vi "Persistent Data to XML.vi"() -> (0 "XML Data":string)   [LabVIEW 2013]
uses:
  Types/Persistent Data.ctl
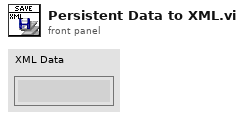
[diagram p1: front panel]
types:
  T1 = typedef "Persistent Data.ctl" = cluster{"File Name":string, "Save Directory":path, "Version":string}
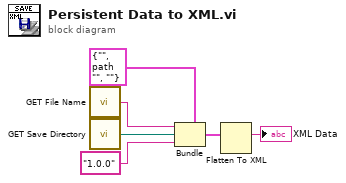
[diagram p0: block diagram]
diagram:
  n1 = call "GET File Name.vi"() -> ("File Name"=w3:string)
  n2 = call "GET Save Directory.vi"() -> ("Save Directory"=w4:path)
  n3 = Bundle(cluster=T1 {"File Name"="", "Save Directory"=path "", "Version"=""} ("Persistent Data"), "File Name"=w3, "Save Directory"=w4, "Version"="1.0.0") -> (w6:T1)
  n4 = Flatten To XML(anything=w6) -> (xml string=→"XML Data":string)
